vi "GMonitor_Feng.vi"(5 "Time Stamp":timestamp, 6 "v1":dbl[](array[numeric]) format="%#_6p", 7 "v0":dbl[](array[numeric]) format="%#_6p", 8 "lockin information":T1, 9 "tdms file":refnum<k34>) -> (0 "FtR":dbl, 1 "FtG":dbl, 2 "TtR":dbl, 3 "TtG":dbl, 4 "tdms file out":refnum<k34>)   [LabVIEW 2013]
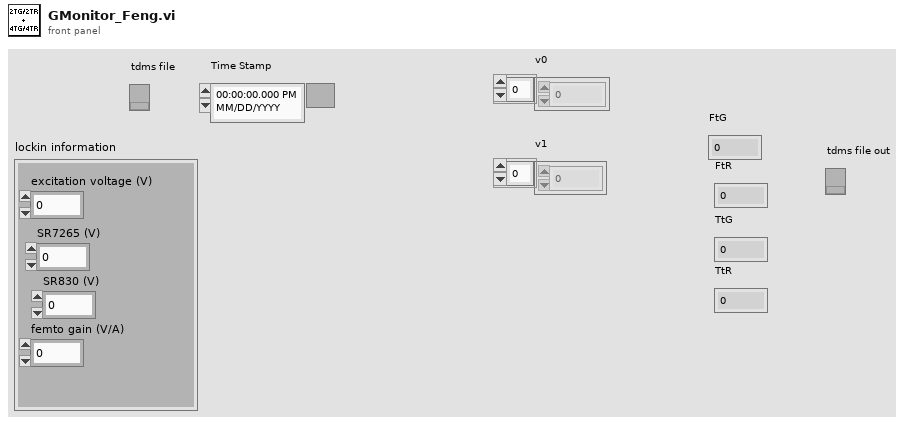
[diagram p1: front panel]
types:
  T1 = cluster{"excitation voltage (V)":dbl, "SR7265 (V)":dbl, "SR830 (V)":dbl, "femto gain (V/A)":dbl}
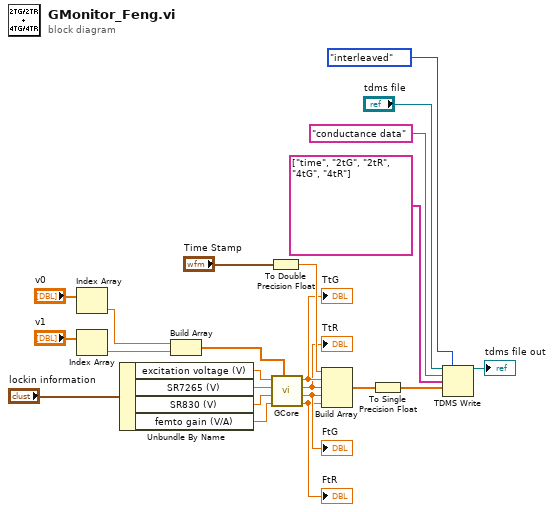
[diagram p0: block diagram]
diagram:
  n1 = Index Array(array="v0") -> (element=w3:dbl)  [unwired: 1 in]
  n2 = Index Array(array="v1") -> (element=w1:dbl)  [unwired: 1 in]
  n3 = Unbundle By Name("lockin information") -> ("excitation voltage (V)"=w12:dbl, "SR7265 (V)"=w11:dbl, "SR830 (V)"=w10:dbl, "femto gain (V/A)"=w9:dbl)
  n4 = Build Array(w3, w1) -> (w14:dbl[])
  n5 = To Double Precision Float(number="Time Stamp") -> (double precision float=w22:dbl)
  n6 = call "GCore.vi"("G data"=w14, "Femto Gain (V/A)"=w9, "SR830 sensitivity"=w10, "SR7265 sensitivity (V)"=w11, "Excitation voltage (V)"=w12) -> ("4tR"=w5:dbl, "4tG"=w6:dbl, "2tR"=w7:dbl, "2tG"=w8:dbl)
  "TtG" <- w8
  "TtR" <- w7
  "FtG" <- w6
  "FtR" <- w5
  n7 = Build Array(w22, w8, w7, w6, w5) -> (w19:dbl[])
  n8 = To Single Precision Float(number=w19) -> (single precision float=w18:sgl[])
  n9 = TDMS Write(0:"tdms file", 1:enum16{"decimated", "interleaved"}."interleaved" ("data layout (0:decimated)"), 5:"conductance data", 7:string[] ["time", "2tG", "2tR", "4tG", "4tR"], 9:w18) -> (4:→"tdms file out":refnum<k34>)  [unwired: 1 in, 3 out]
